vi "SAOMM-ROI-Stats.vi"(5 "ImageBuffer":u16[][](array[numeric]), 9 "ObjectMask":u8[][](array[numeric]), 12 "intervals":i32=10) -> (6 "ROI Histogram":T1(graph), 10 "ImageStat":T2 {"SNR" format="%0.2f"; "mean" format="%0.2f"; "Flux" format="%0.2f"; "Variance" format="%0.2f"; "median" format="%0.2f"})   [LabVIEW 2019]
uses:
  <vilib>/Analysis/NI_AALBase.lvlib
panel:
  out "Noise":dbl
  out "Signal":dbl
  out "BackGnd Variance":dbl format="%0.2f"
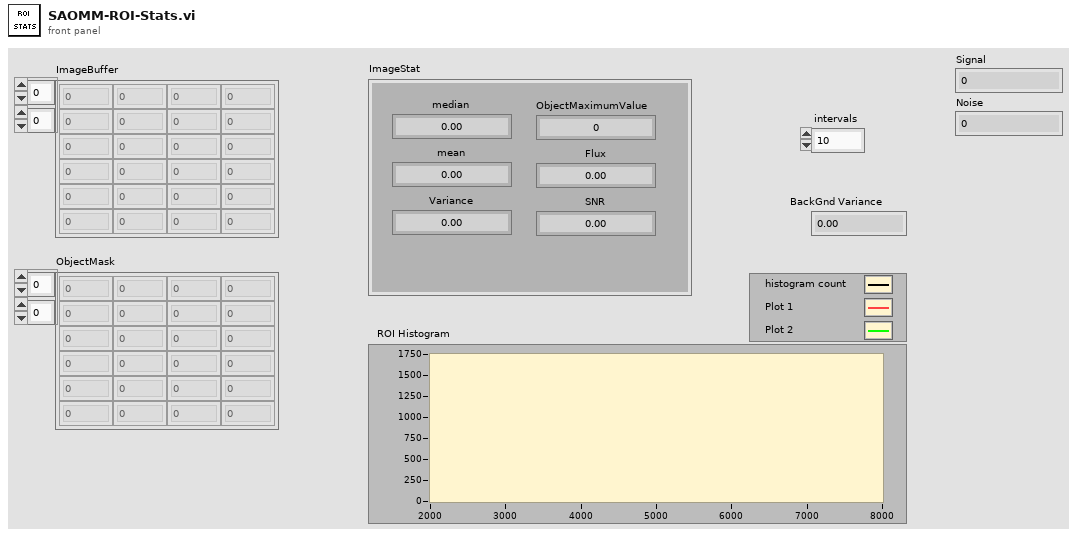
[diagram p1: front panel]
types:
  T1 = cluster{"X Values":dbl[], "Histogram: h(x)":i32[]}[]
  T2 = cluster{"median":dbl, "mean":dbl, "Variance":dbl, "ObjectMaximumValue":dbl, "Flux":dbl, "SNR":dbl}
  T3 = cluster{"X Values":dbl[], "Histogram: h(x)":i32[]}
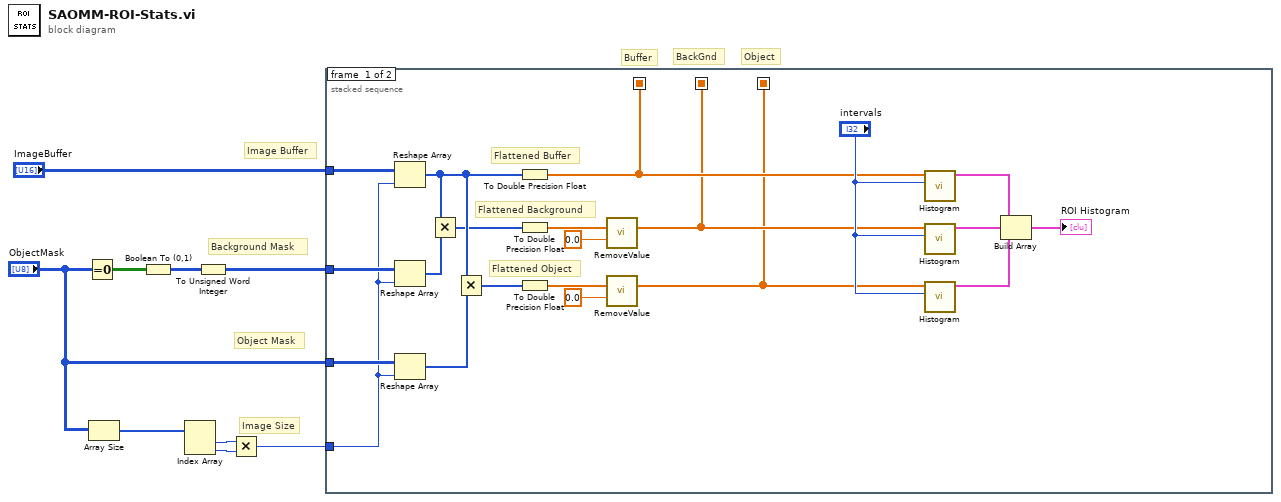
[diagram p0: block diagram]
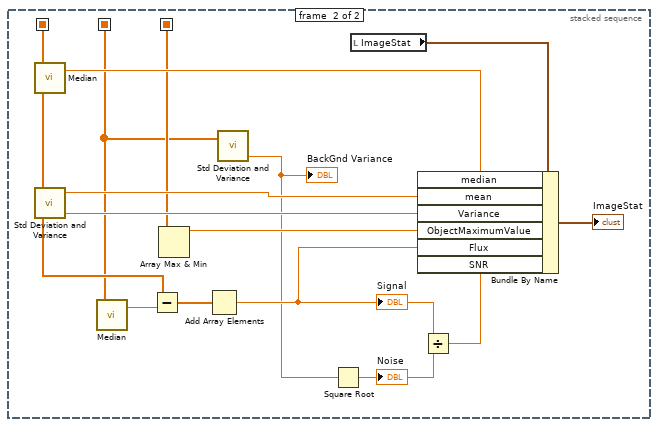
[diagram p2: hidden frame]
diagram:
  # "Object"
  # "BackGnd"
  # "Buffer"
  # "Image Size"
  # "Image Buffer"
  # "Object Mask"
  # "Background Mask"
  n1 = Equal To 0?(x="ObjectMask") -> (x = 0?=w9:bool[][])
  n2 = Array Size(array="ObjectMask") -> (size(s)=w7:i32[])
  n3 = Boolean To (0,1)(Boolean=w9) -> (0, 1=w8:i16[][])
  n4 = Index Array(array=w7) -> (element #1=w6:i32, element #2=w5:i32)  [unwired: 2 in]
  n5 = To Unsigned Word Integer(number=w8) -> (unsigned 16bit integer=w1:u16[][])
  n6 = Multiply(x=w6, y=w5) -> (x*y=w3:i32)
  n7 = stacked-sequence {
    seq-local: [w12 _] -> [_ w38]
    seq-local: [w11 _] -> [_ w36]
    seq-local: [w10 _] -> [_ w40]
    tunnel: "ImageBuffer" -> [w30 _]
    tunnel: w1 -> [w29 _]
    tunnel: "ObjectMask" -> [w28 _]
    tunnel: w3 -> [w26 _]
    frame #0 {
      # "Flattened Object"
      # "Flattened Background"
      # "Flattened Buffer"
      n8 = Reshape Array(w30, w26) -> (w24:u16[])
      n9 = Reshape Array(w29, w26) -> (w27:u16[])
      n10 = Reshape Array(w28, w26) -> (w25:u8[])
      n11 = Multiply(x=w24, y=w27) -> (x*y=w22:u16[])
      n12 = Multiply(x=w24, y=w25) -> (x*y=w23:u16[])
      n13 = To Double Precision Float(number=w24) -> (double precision float=w12:dbl[])
      n14 = To Double Precision Float(number=w22) -> (double precision float=w21:dbl[])
      n15 = To Double Precision Float(number=w23) -> (double precision float=w20:dbl[])
      n16 = call "RemoveValue.vi"("Input aArray"=w21, "Valeur à enlever"=0.0) -> ("Output Array"=w11:dbl[])  [unwired: 13 in]
      n17 = call "RemoveValue.vi"("Input aArray"=w20, "Valeur à enlever"=0.0) -> ("Output Array"=w10:dbl[])  [unwired: 13 in]
      n18 = call <vilib>:"Histogram.vi"("intervals"="intervals", "X"=w12) -> ("Histogram Graph"=w16:T3)  [unwired: 6 in, 3 out]
      n19 = call <vilib>:"Histogram.vi"("intervals"="intervals", "X"=w11) -> ("Histogram Graph"=w14:T3)  [unwired: 6 in, 3 out]
      n20 = call <vilib>:"Histogram.vi"("intervals"="intervals", "X"=w10) -> ("Histogram Graph"=w15:T3)  [unwired: 6 in, 3 out]
      n21 = Build Array(w16, w14, w15) -> (→"ROI Histogram":T1)
    }
    frame #1 {
      n22 = call <vilib>:"Median.vi"("X"=w38) -> ("median"=w43:dbl)  [unwired: 1 out]
      n23 = call <vilib>:"Std Deviation and Variance.vi"("X"=w38) -> ("mean"=w42:dbl, "variance"=w41:dbl)  [unwired: 1 in, 1 out]
      n24 = call <vilib>:"Median.vi"("X"=w36) -> ("median"=w34:dbl)  [unwired: 1 out]
      n25 = Subtract(x=w38, y=w34) -> (x-y=w37:dbl[])
      n26 = Array Max & Min(array=w40) -> (max value=w39:dbl)  [unwired: 3 out]
      n27 = Add Array Elements(numeric array=w37) -> (sum=w33:dbl)
      "Signal" <- w33
      n28 = call <vilib>:"Std Deviation and Variance.vi"("X"=w36) -> ("variance"=w31:dbl)  [unwired: 1 in, 2 out]
      "BackGnd Variance" <- w31
      n29 = Square Root(x=w31) -> (sqrt(x)=w32:dbl)
      "Noise" <- w32
      n30 = local read "ImageStat"() -> (w45:T2)
      n31 = Divide(x=w33, y=w32) -> (x/y=w35:dbl)
      n32 = Bundle By Name(cluster=w45, "median"=w43, "mean"=w42, "Variance"=w41, "ObjectMaximumValue"=w39, "Flux"=w33, "SNR"=w35) -> (→"ImageStat":T2)
    }
  }
